vi "ROI entry-Event handler-Clear All ROI.vi"   [LabVIEW 2013]
uses:
  Typedefs/ROI management FG states.ctl
types:
  T1 = typedef "ROI management FG states.ctl" = enum16{"Read", "Write", "Clear Last", "Clear All", "Update ROIs time", "Reload last ROI set", "Offset all ROI", "Offset visible ROI"}
  T2 = typedef "ROI ID Enum.ctl" = enum16{"Point", "MiniScan", "Comp. MiniScan", "Rectangle", "Comp. volume", "Arb. plane point"}
  T3 = typedef "ROI parameters data type.ctl" = cluster{"ROI index":dbl, "ROI ID":dbl, "ROI Time (ns)":dbl, "Pixels in ROI":dbl, "X start":dbl, "Y start":dbl, "Z start":dbl, "X stop":dbl, "Y stop":dbl, "Z stop":dbl, "Angle (deg)":dbl, "Composite ID":dbl, "Number of lines":dbl, "Frame Size":dbl, "Zoom":dbl, "Laser Power (%)":dbl, "ROI group ID":dbl}
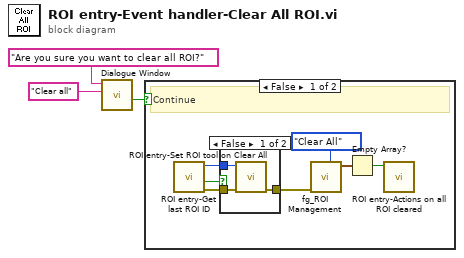
[diagram p0: block diagram]
diagram:
  n1 = call "Dialogue Window.vi"("Caption-Right button (OK)"="Clear all" ("T button name (\"OK\")"), "Message string"="Are you sure you want to clear all ROI?" ("message")) -> ("Cancelled (Left button pressed)"=w3:bool)  [unwired: 7 in, 2 out]
  n2 = case shown="False" w3 {
    frame False {
      # "Continue"
      n3 = call "ROI entry-Get last ROI ID.vi"() -> ("error out"=w5:errorcluster, "NO ROI"=w4:bool, "ROI ID Enum"=w6:T2)  [unwired: 8 in, 1 out]
      n4 = case shown="False" w4 {
        tunnel: [w13 w14] -> w7
        tunnel: w6 -> [w12 _]
        tunnel: w5 -> [w11 w14]
        frame False {
          n5 = call "ROI entry-Set ROI tool on Clear All.vi"("error in (no error)"=w11, "Last ROI ID Enum"=w12) -> ("error out"=w13:errorcluster)  [unwired: 9 in]
        }
        frame True {
        }
      }
      n6 = call "fg_ROI Management.vi"("Function"=ROI_management_FG_states."Clear All", "error in (no error)"=w7) -> ("ROI Setup"=w9:T3[])  [unwired: 5 in, 4 out]
      n7 = Empty Array?(array=w9) -> (empty?=w10:bool)
      n8 = call "ROI entry-Actions on all ROI cleared.vi"("No ROIs (T)"=w10) -> ()  [unwired: 11 in]
    }
    frame True {
      # "Cancelled"
    }
  }
